vi "Featire detect shift method.vi"(0 "Xvalues":dbl[](array[numeric]), 1 "Yvalues":dbl[](array[numeric]), 3 "magnitude  limit":i32, 4 "Shift":i32=-20, 5 "Window":i32=2 min=2 step=2) -> (14 "Feature positions":dbl[](array[numeric]), 15 "Feature ampltuides":dbl[](array[numeric]))   [LabVIEW 2014]
uses:
  <vilib>/ptbypt/NI_PtbyPt.lvlib
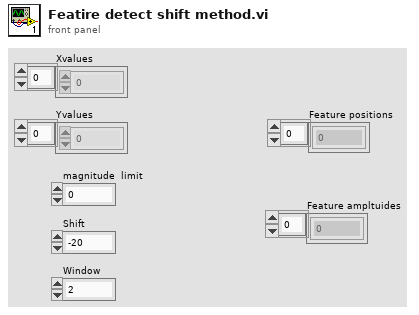
[diagram p1: front panel]
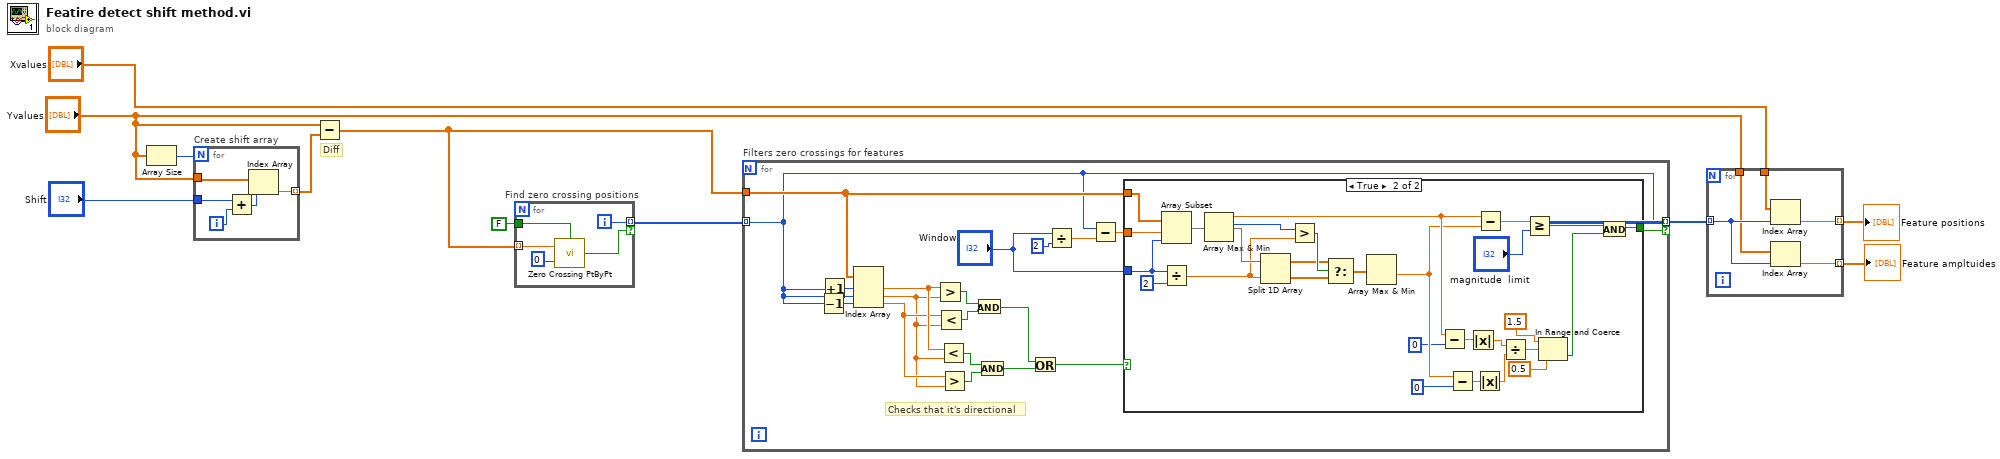
[diagram p0: block diagram]
diagram:
  # "Diff"
  n1 = Array Size(array="Yvalues") -> (size(s)=w11:i32)
  n2 = for "Create shift array" {
    N: w11 -> [_]
    tunnel: "Yvalues" -> [w16]
    tunnel: [w13] -> w10 mode=indexing
    tunnel: "Shift" -> [w12]
    i -> [w15]
    n3 = Add(x=w12, y=w15) -> (x+y=w14:i32)
    n4 = Index Array(array=w16, index=w14) -> (element=w13:dbl)
  }
  n5 = Subtract(x="Yvalues", y=w10) -> (x-y=w8:dbl[])
  n6 = for "Find zero crossing positions" {
    tunnel: w8 -> [w21] mode=indexing
    tunnel: FALSE -> [w20]
    tunnel: [w18] -> w4 mode=indexing if=w17
    i -> [w18]
    n7 = call <vilib>:"Zero Crossing PtByPt.vi"("initialize"=w20, "direction"=0, "input data point"=w21) -> ("crossing"=w17:bool)
  }
  n8 = for "Filters zero crossings for features" {
    tunnel: w8 -> [w31]
    tunnel: w4 -> [w22] mode=indexing
    tunnel: [w22] -> w3 mode=indexing if=w34
    # "Checks that it's directional"
    n9 = Decrement(x=w22) -> (x-1=w32:i32)
    n10 = Increment(x=w22) -> (x+1=w33:i32)
    n11 = Index Array(array=w31, index #1=w33, index #2=w22, index #3=w32) -> (element #1=w28:dbl, element #2=w25:dbl, element #3=w27:dbl)
    n12 = Greater?(x=w28, y=w25) -> (0:w40:bool)
    n13 = Less?(x=w27, y=w25) -> (x < y?=w39:bool)
    n14 = Less?(x=w28, y=w25) -> (x < y?=w38:bool)
    n15 = Greater?(x=w27, y=w25) -> (0:w37:bool)
    n16 = And(x=w40, y=w39) -> (x .and. y?=w36:bool)
    n17 = And(x=w38, y=w37) -> (x .and. y?=w35:bool)
    n18 = Or(x=w36, y=w35) -> (x .or. y?=w26:bool)
    n19 = Divide(x="Window", y=2) -> (x/y=w23:dbl)
    n20 = Subtract(x=w22, y=w23) -> (x-y=w29:dbl)
    n21 = case shown="True" w26 {
      selector: w26 -> [w41 _]
      tunnel: [w41 w46] -> w34
      tunnel: w31 -> [_ w66]
      tunnel: w29 -> [_ w65]
      tunnel: "Window" -> [_ w63]
      frame False {
      }
      frame True {
        n22 = Array Subset(array=w66, index=w65, length=w63) -> (w64:dbl[])
        n23 = Divide(x=w63, y=2) -> (x/y=w60:dbl)
        n24 = Array Max & Min(array=w64) -> (max value=w55:dbl, max index (indices)=w61:i32)  [unwired: 2 out]
        n25 = Split 1D Array(array=w64, index=w60) -> (first subarray=w58:dbl[], second subarray=w57:dbl[])
        n26 = Greater?(x=w61, y=w60) -> (0:w59:bool)
        n27 = Select(t=w58, s=w59, f=w57) -> (s? t:f=w56:dbl[])
        n28 = Array Max & Min(array=w56) -> (min value=w54:dbl)  [unwired: 3 out]
        n29 = Subtract(x=w55, y=0) -> (x-y=w53:dbl)
        n30 = Subtract(x=w54, y=0) -> (x-y=w52:dbl)
        n31 = Absolute Value(x=w53) -> (abs(x)=w51:dbl)
        n32 = Absolute Value(x=w52) -> (abs(x)=w50:dbl)
        n33 = Subtract(x=w55, y=w54) -> (x-y=w68:dbl)
        n34 = Divide(x=w51, y=w50) -> (x/y=w49:dbl)
        n35 = Greater Or Equal?(x=w68, y="magnitude  limit") -> (x >= y?=w45:bool)
        n36 = In Range and Coerce(upper limit=1.5, x=w49, lower limit=0.5) -> (In Range?=w44:bool)  [unwired: 1 out]
        n37 = And(x=w45, y=w44) -> (x .and. y?=w46:bool)
      }
    }
  }
  n38 = for {
    tunnel: w3 -> [w71] mode=indexing
    tunnel: "Xvalues" -> [w72]
    tunnel: [w73] -> w1 mode=indexing
    tunnel: "Yvalues" -> [w70]
    tunnel: [w69] -> w2 mode=indexing
    n39 = Index Array(array=w72, index=w71) -> (element=w73:dbl)
    n40 = Index Array(array=w70, index=w71) -> (element=w69:dbl)
  }
  "Feature positions" <- w1
  "Feature ampltuides" <- w2
